vi "Read Description.vi"(11 "Whip in":refnum<class "Whip.lvclass">) -> (2 "Description":string, 3 "Whip out":refnum<class "Whip.lvclass">)   [LabVIEW 2020, in "Whip.lvclass"]
uses:
  Whip.lvclass
  Whip.lvclass/Whip.ctl
  Beverage.lvclass
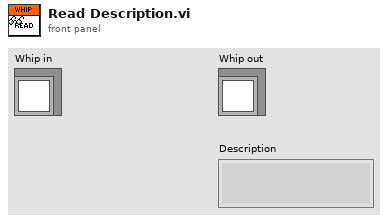
[diagram p1: front panel]
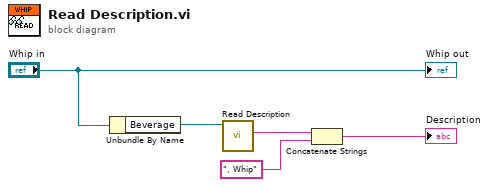
[diagram p0: block diagram]
diagram:
  n1 = Unbundle By Name("Whip in") -> ("Beverage"=w4:refnum<class "Beverage.lvclass">)
  n2 = call-dynamic "Read Description.vi"("Beverage in"=w4) -> ("Description"=w3:string)  [unwired: 9 in, 1 out]
  n3 = Concatenate Strings(w3, ", Whip" ("string")) -> (→"Description":string)
  "Whip out" <- "Whip in"
